vi "Receive Response.vi"(8 "error in":errorcluster, 10 "Command in":T1, 11 "Kronos in":refnum<class "Kronos.lvclass">) -> (0 "error out":errorcluster, 3 "Kronos out":refnum<class "Kronos.lvclass">)   [LabVIEW 2018, in "Kronos.lvlib" / "Kronos.lvclass"]
doc: "Read response data from laser"
uses:
  Kronos.lvclass
  PPLs/Laser/Parent/Laser.lvlibp/Custom Controls/Command List.ctl
  <vilib>/Utility/error.llb/whitespace.ctl
  PPLs/Laser/Parent/Laser.lvlibp/Laser.lvclass
  C:/AME Test Engineering/LabVIEW/PPLs/Laser/Parent/Laser.lvlibp/Laser.lvclass
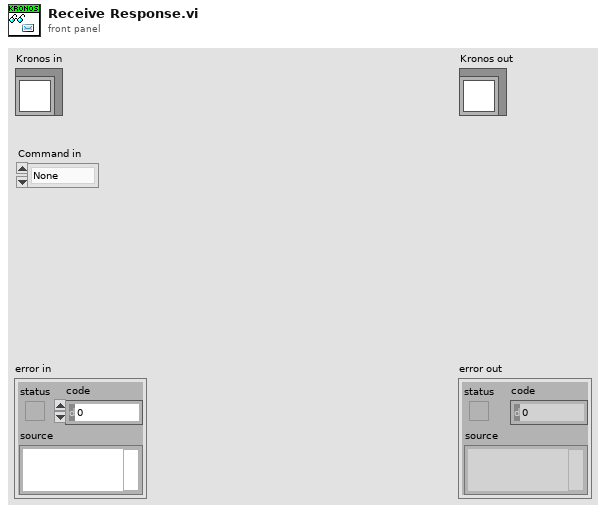
[diagram p1: front panel]
types:
  T1 = typedef "Laser.lvlibp/Laser.lvclass/Command List.ctl" = enum16{"None", "Config?", "Volt?", "ThCase?", "STS?", "Mon?", "Help?", "HB", "Verbose", "Spnt", "Ext", "PRF", "Start", "Stop", "PRF?", "State?", "Status?", "Stat?", "Read HB", "Logon", "Poutmax", "saveconfig", "Reset", "Poutmax?", "PoutCommandMax", "PoutCommandMax?", "FreqMin", "FreqMin?"}
  T2 = typedef "whitespace.ctl" = u16
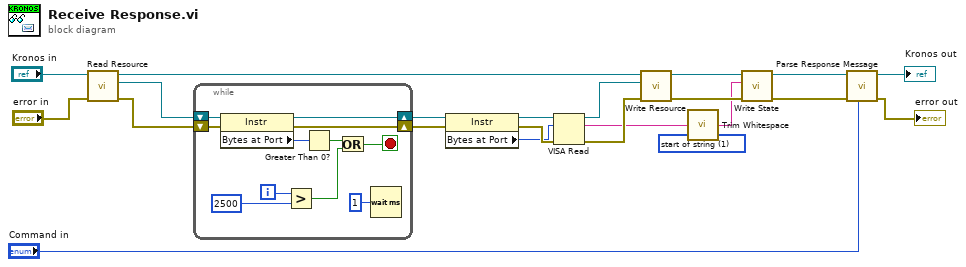
[diagram p0: block diagram]
diagram:
  w1 = T2 1 items=["both", "start of string", "end of string"] ("location (both)")
  n1 = call "Read Resource.vi"("error in (no error)"="error in", "Laser in"="Kronos in") -> ("error out"=w10:errorcluster, "Resource"=w9:refnum<visa-resource-name>, "Laser out"=w17:refnum<class "Kronos.lvclass">)  [unwired: 7 in]
  n2 = while {
    shift-right: [w26] -> w14
    shift-left: w9 -> [w33]
    shift-right: [w25] -> w18
    shift-left: w10 -> [w24]
    i -> [w30]
    stop <- w27 stop-if-true
    n3 = property class="Instr"(reference=w33, error in=w24) -> (reference out=w26:refnum<visa-resource-name>, error out=w25:errorcluster, "Bytes at Port"=w32:u32)
    n4 = Greater?(x=w30, y=2500) -> (0:w28:bool)
    n5 = Greater Than 0?(x=w32) -> (x > 0?=w31:bool)
    n6 = Or(x=w31, y=w28) -> (x .or. y?=w27:bool)
    n7 = Wait (ms)(milliseconds to wait=u32 1) -> ()  [unwired: 1 out]
  }
  n8 = property class="Instr"(reference=w14, error in=w18) -> (reference out=w13:refnum<visa-resource-name>, error out=w12:errorcluster, "Bytes at Port"=w11:u32)
  n9 = VISA Read(VISA resource name=w13, byte count=w11, error in (no error)=w12) -> (VISA resource name out=w15:refnum<visa-resource-name>, read buffer=w3:string, error out=w16:errorcluster)  [unwired: 1 out]
  n10 = call "Write Resource.vi"("error in (no error)"=w16, "Resource"=w15, "Laser in"=w17) -> ("error out"=w20:errorcluster, "Laser out"=w19:refnum<class "Kronos.lvclass">)  [unwired: 7 in]
  n11 = call <vilib>:"Trim Whitespace.vi"("string"=w3, "location (both)"=w1) -> ("trimmed string"=w2:string)
  n12 = call "Write State.vi"("error in (no error)"=w20, "State"=w2, "Laser in"=w19) -> ("error out"=w21:errorcluster, "Laser out"=w22:refnum<class "Kronos.lvclass">)  [unwired: 7 in]
  n13 = call "Parse Response Message.vi"("Command in"="Command in", "error in"=w21, "Kronos in"=w22) -> ("error out"=→"error out":errorcluster, "Kronos out"=→"Kronos out":refnum<class "Kronos.lvclass">)  [unwired: 7 in]
